vi "Resize.vi"(9 "Container State":T1, 11 "Display State In":T2) -> ()   [LabVIEW 2019, in "ExpandVertical.xctl"]
uses:
  ExpandVertical.xctl
  State.ctl
  <vilib>/_xctls/Container State.ctl
  <vilib>/Utility/miscctls.llb/LVPointTypeDef.ctl
  <vilib>/_xctls/XControlSupport.lvlib
panel:
  out "error out":errorcluster
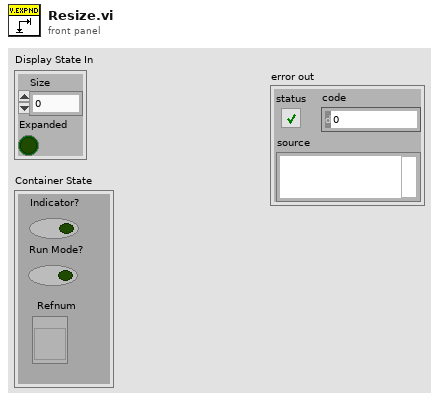
[diagram p1: front panel]
types:
  T1 = typedef "XControlSupport.lvlib/Container State.ctl" = cluster{"Indicator?":bool, "Run Mode?":bool, " Refnum":refnum<vi>}
  T2 = typedef "ExpandVertical.xctl/State.ctl" = cluster{"Size":i16, "Expanded":bool}
  T3 = enum16{"Always On", "Always Off", "Off While Running"}
  T4 = typedef "LVPointTypeDef.ctl" = cluster{"Horizontal":i16, "Vertical":i16}
  T5 = typedef "LVRectTypeDef.ctl" = cluster{"Left":i16, "Top":i16, "Right":i16, "Bottom":i16}
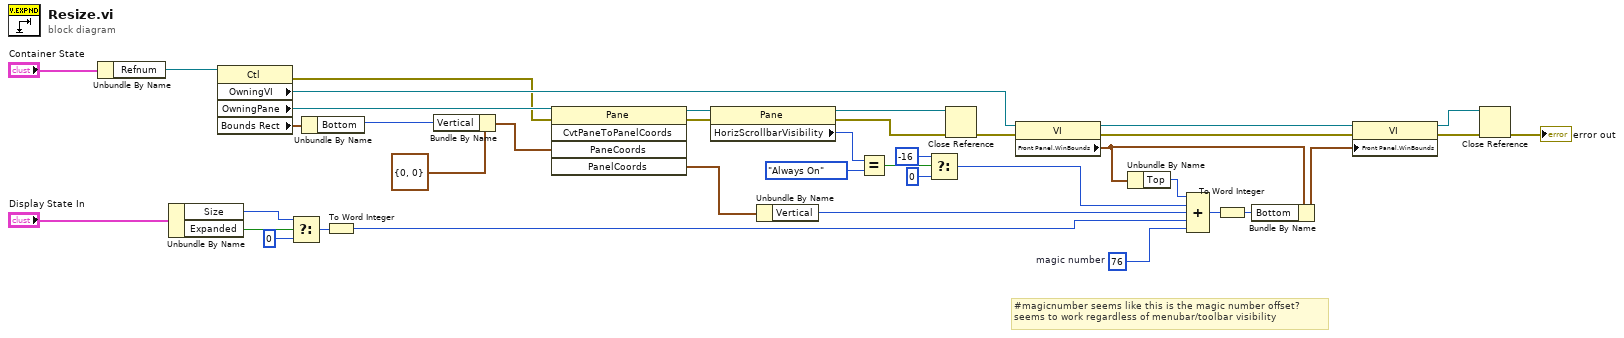
[diagram p0: block diagram]
diagram:
  w1 = i16 76  # magic number
  # "#magicnumber seems like this is the magic number offset?\nseems to work regardless of menubar/toolbar visibility"
  n1 = Unbundle By Name("Container State") -> ("Refnum"=w37:refnum<vi>)
  n2 = Unbundle By Name("Display State In") -> ("Size"=w34:i16, "Expanded"=w35:bool)
  n3 = property class="Ctl"(reference=w37) -> (error out=w15:errorcluster, "OwningVI"=w23:refnum<vi>, "OwningPane"=w16:refnum<vi>, "Bounds Rect"=w21:T5)  [unwired: 1 in, 1 out]
  n4 = Select(t=w34, s=w35, f=i16 0) -> (s? t:f=w33:i16)
  n5 = Unbundle By Name(w21) -> ("Bottom"=w17:i16)
  n6 = To Word Integer(number=w33) -> (16bit integer=w2:i16)
  n7 = Bundle By Name(cluster=T4 {"Horizontal"=0, "Vertical"=0} ("Pane Coordinates"), "Vertical"=w17) -> (w18:T4)
  n8 = invoke class="Pane" method="CvtPaneToPanelCoords"(reference=w16, error in=w15, "PaneCoords"=w18) -> (reference out=w10:refnum<vi>, error out=w14:errorcluster, "PanelCoords"=w12:T4)  [unwired: 2 in, 2 out]
  n9 = property class="Pane"(reference=w10, error in=w14) -> (reference out=w9:refnum<vi>, error out=w11:errorcluster, "HorizScrollbarVisibility"=w8:T3)
  n10 = Unbundle By Name(w12) -> ("Vertical"=w20:i16)
  n11 = Equal?(x=w8, y=T3."Always On") -> (x = y?=w6:bool)
  n12 = Select(t=i16 -16, s=w6, f=i16 0) -> (s? t:f=w3:i16)
  n13 = Close Reference(reference=w9, error in (no error)=w11) -> (error out=w13:errorcluster)
  n14 = property class="VI"(reference=w23, error in=w13) -> (reference out=w22:refnum<vi>, error out=w28:errorcluster, "Front Panel.WinBounds"=w25:T5)
  n15 = Unbundle By Name(w25) -> ("Top"=w24:i16)
  n16 = Compound Arithmetic op=ADD(w24, w3, w20, w2, w1) -> (w39:i16)
  n17 = To Word Integer(number=w39) -> (16bit integer=w26:i16)
  n18 = Bundle By Name(cluster=w25, "Bottom"=w26) -> (w29:T5)
  n19 = property class="VI"(reference=w22, error in=w28, "Front Panel.WinBounds"=w29) -> (reference out=w31:refnum<vi>, error out=w30:errorcluster)
  n20 = Close Reference(reference=w31, error in (no error)=w30) -> (error out=→"error out":errorcluster)
